vi "Epoch Factory.vi"(11 "Epoch (Local System)":T1=enum."Unix") -> (3 "Epoch object":refnum<class "Epoch.lvclass">)   [LabVIEW 2018]
uses:
  <vilib>/LabVIEW Open Source Project/Epoch Date & Time/epoch/Epoch.lvclass
  <vilib>/LabVIEW Open Source Project/Epoch Date & Time/Epochs -- enum.ctl
  <vilib>/LabVIEW Open Source Project/Epoch Date & Time/epoch.UTC/Epoch.UTC.lvclass
  C:/Program Files (x86)/National Instruments/LabVIEW 2018/vi.lib/LabVIEW Open Source Project/Epoch Date & Time/epoch/Epoch.lvclass
  <vilib>/LabVIEW Open Source Project/Epoch Date & Time/epoch.UNIX/Epoch.UNIX.lvclass
  <vilib>/LabVIEW Open Source Project/Epoch Date & Time/epoch.GPS/Epoch.GPS.lvclass
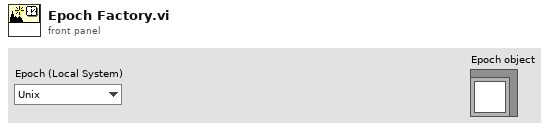
[diagram p1: front panel]
types:
  T1 = typedef "Epochs -- enum.ctl" = enum16{"Local", "UTC", "Unix", "GPS"}
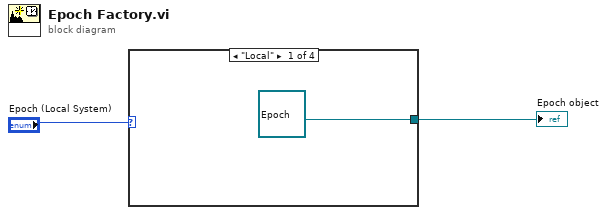
[diagram p0: block diagram]
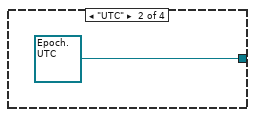
[diagram p2: hidden frame]
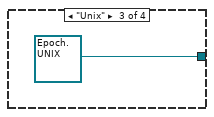
[diagram p3: hidden frame]
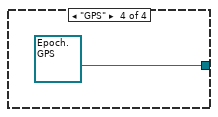
[diagram p4: hidden frame]
diagram:
  n1 = case shown="\"Local\"" "Epoch (Local System)" {
    tunnel: [refnum<class "Epoch.lvclass"> refnum ("Epoch.lvclass") refnum<class "Epoch.UTC.lvclass"> refnum ("Epoch.UTC.lvclass") refnum<class "Epoch.UNIX.lvclass"> refnum ("Epoch.UNIX.lvclass") refnum<class "Epoch.GPS.lvclass"> refnum ("Epoch.GPS.lvclass")] -> w1
    frame "Local" {
    }
    frame "UTC" {
    }
    frame "Unix" {
    }
    frame "GPS" {
    }
  }
  "Epoch object" <- w1
